vi "Drive.SetSpeedDem.vi"(10 "RSpeedDemand (ft/s)":dbl, 11 "LSpeedDemand (ft/s)":dbl) -> ()   [LabVIEW 2020]
doc: "set speed demand variable for drive (called in human)"
uses:
  Drive.Global.vi
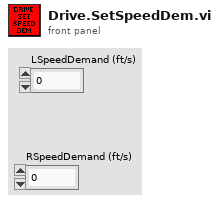
[diagram p1: front panel]
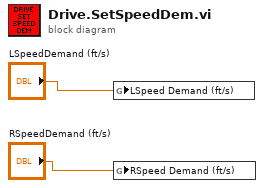
[diagram p0: block diagram]
diagram:
  n1 = global write "Drive.Global.vi" "LSpeed Demand (ft/s)"("LSpeedDemand (ft/s)") -> ()
  n2 = global write "Drive.Global.vi" "RSpeed Demand (ft/s)"("RSpeedDemand (ft/s)") -> ()
